vi "Test Archiver.vi"() -> ()   [LabVIEW 2019]
uses:
  Settings/Setting Database/Typedefs/PublicEvents--Setting Database.PathsUpdated.ctl
  Settings/Path Settings/Path Settings.lvclass
  C:/Users/Albro/Documents/GitHub/AFM-Lithography/lvsrc/Classes/Settings/ObjectSettings/ObjectSettings.lvclass
  Settings/Setting Database/Typedefs/PublicEvents--Setting Database.RectanglesUpdated.ctl
  Settings/Rectangle Settings/Rectangle Settings.lvclass
  Settings/Setting Database/Typedefs/PublicEvents--Setting Database.FunnelsUpdated.ctl
  Settings/Funnel Settings/Funnel Settings.lvclass
  Settings/Setting Database/Typedefs/PublicEvents--Setting Database.DotsUpdated.ctl
  Settings/Dot Settings/Dot Settings.lvclass
  Settings/Setting Database/Setting Database.lvclass
  C:/Program Files (x86)/National Instruments/LabVIEW 2019/vi.lib/JKI/JKI SMO/SMO/SMO.lvclass
  <vilib>/JKI/JKI SMO/SMO/SMO.lvclass/SMO.ctl
  <vilib>/JKI/JKI SMO/SMO/Typedefs/SMOState --Enum.ctl
  <vilib>/JKI/JKI SMO/SMO/Private/ReftoDVR--SMO.vi
  <vilib>/addons/_JKI Toolkits/Caraya/classes/Test/Test.lvclass
  <vilib>/addons/_JKI Toolkits/Caraya/classes/Assert/Assert.lvclass
  <vilib>/addons/_JKI Toolkits/Caraya/classes/Assert/Assert Equal Value_Variant.vi
  Archivist.lvclass
  <vilib>/JKI/JKI SMO/SMO/SMO.lvclass
panel:
  out "Numeric":i32
  out "GUIDs 6":string[](array[string])
  out "GUIDs 5":string[](array[string])
  out "GUIDs 4":string[](array[string])
  out "GUIDs 3":string[](array[string])
  out "GUIDs 2":string[](array[string])
  out "GUIDs":string[](array[string])
  out "number of events discarded":u32
  out "error out 2":errorcluster
  out "error out":errorcluster
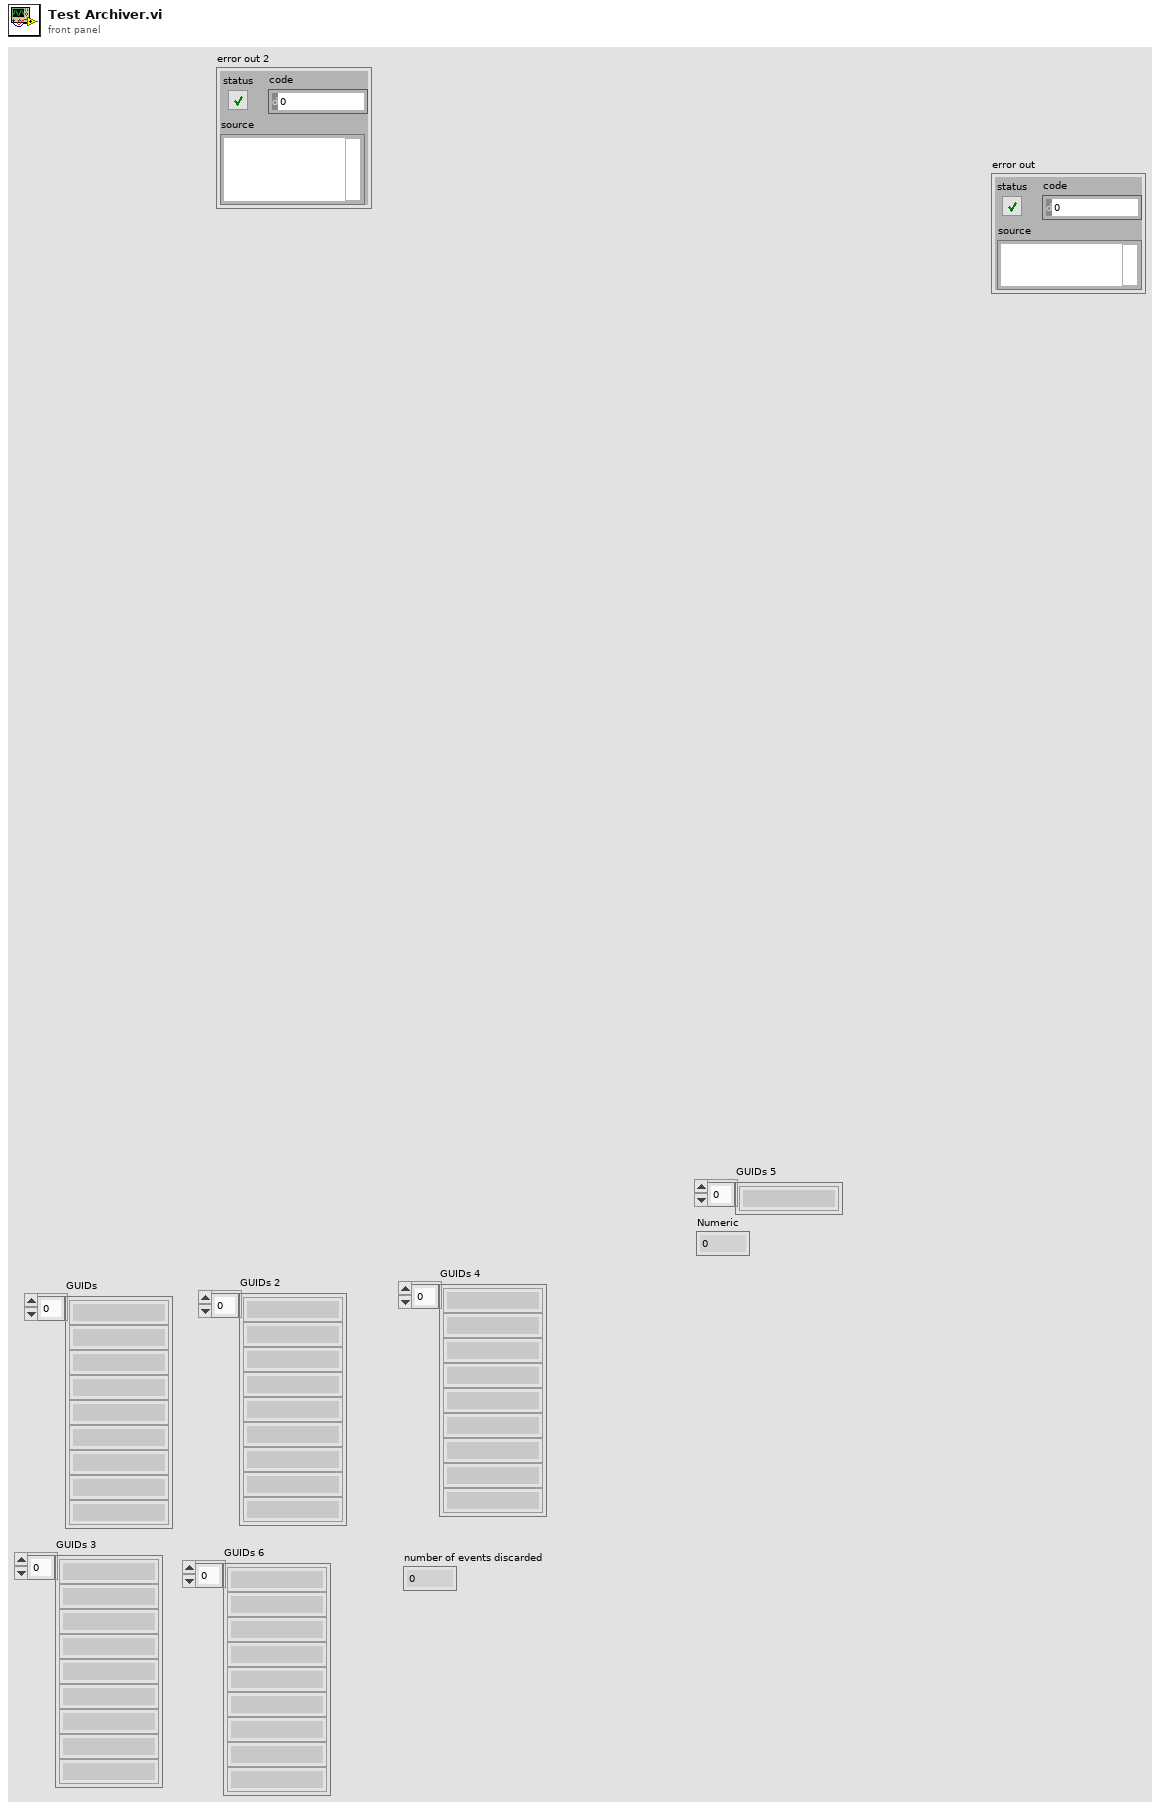
[diagram p1: front panel]
types:
  T1 = typedef "Setting Database.lvclass/PublicEvents--Setting Database.PathsUpdated.ctl" = refnum<class "Path Settings.lvclass">[]
  T2 = typedef "Setting Database.lvclass/PublicEvents--Setting Database.RectanglesUpdated.ctl" = refnum<class "Rectangle Settings.lvclass">[]
  T3 = typedef "Setting Database.lvclass/PublicEvents--Setting Database.FunnelsUpdated.ctl" = refnum<class "Funnel Settings.lvclass">[]
  T4 = typedef "Setting Database.lvclass/PublicEvents--Setting Database.DotsUpdated.ctl" = refnum<class "Dot Settings.lvclass">[]
  T5 = cluster{"Paths":T1, "Rectangles":T2, "Funnels":T3, "Dots":T4}
  T6 = typedef "Setting Database.lvclass/PublicEvents--Cluster.ctl" = cluster{"NewActivePath":refnum<user-event>, "PathsUpdated":refnum<user-event>, "RectanglesUpdated":refnum<user-event>, "NewActiveRectangle":refnum<user-event>, "NewActiveFunnel":refnum<user-event>, "FunnelsUpdated":refnum<user-event>, "NewActiveDot":refnum<user-event>, "DotsUpdated":refnum<user-event>}
  T7 = typedef "SMO.lvclass/Public Events.ctl" = cluster{"Error":refnum<user-event>, "State":refnum<user-event>, "Reserve State":refnum<user-event>}
  T8 = cluster{"Event Registration Refnum":refnum<event-registration>}
  T9 = typedef "SMO.lvclass/SMOState --Enum.ctl" = enum16{"unknown", "Created", "Started", "Stopped"}
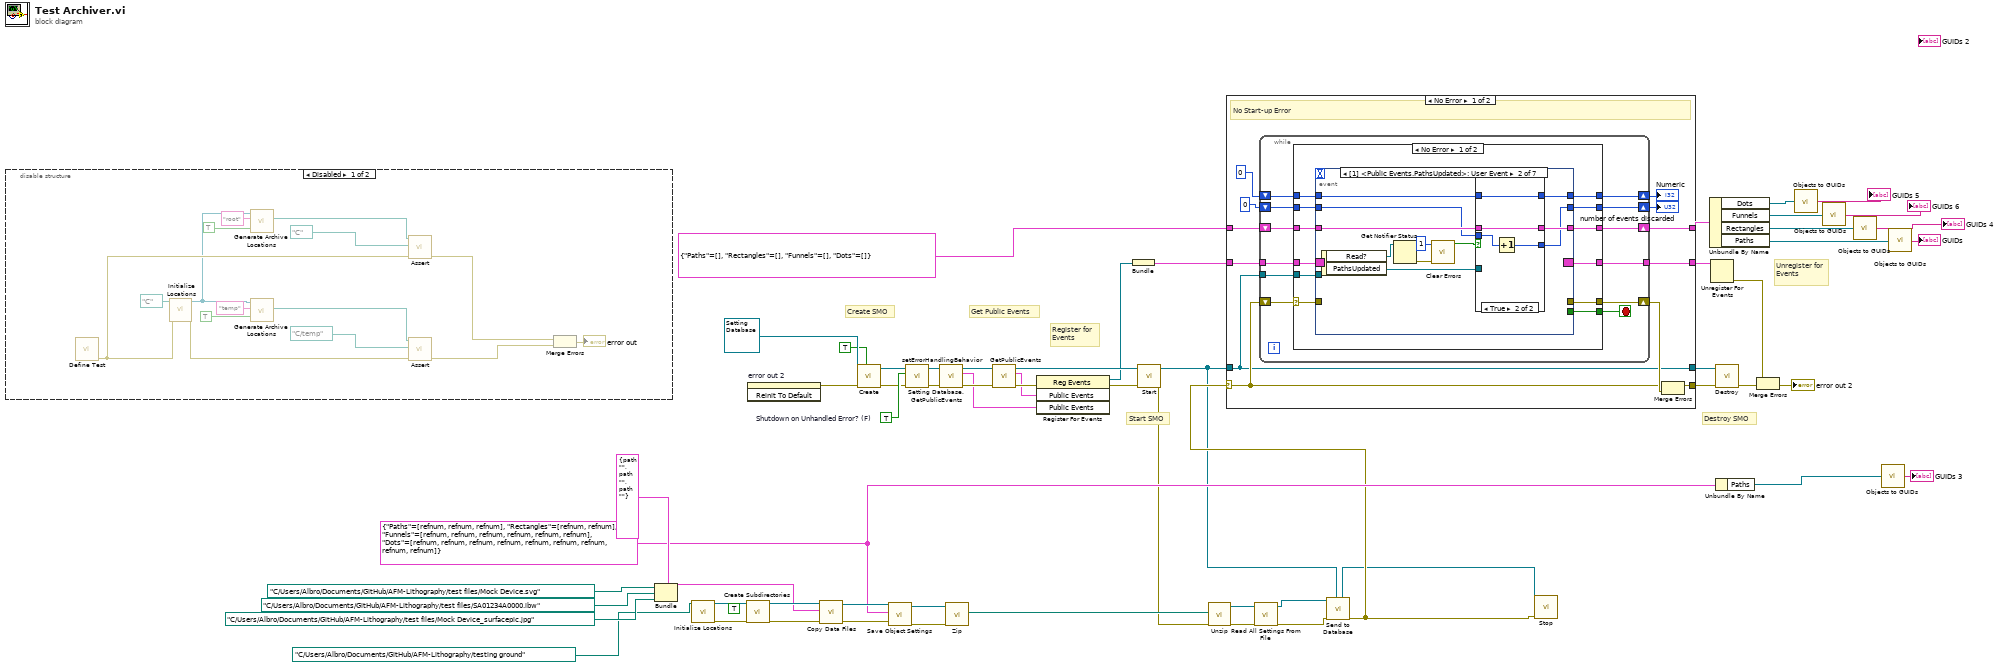
[diagram p0: block diagram]
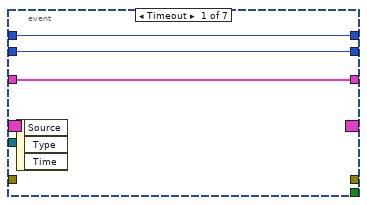
[diagram p2: hidden frame]
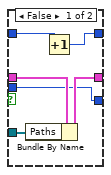
[diagram p3: hidden frame]
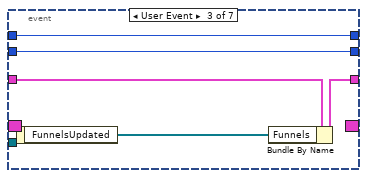
[diagram p4: hidden frame]
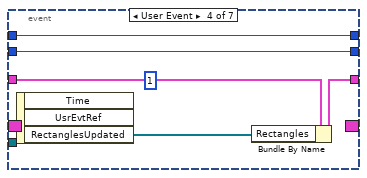
[diagram p5: hidden frame]
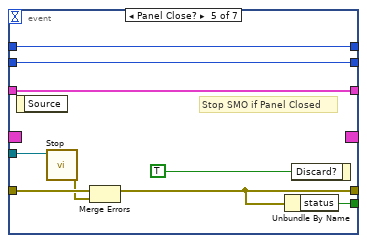
[diagram p6: hidden frame]
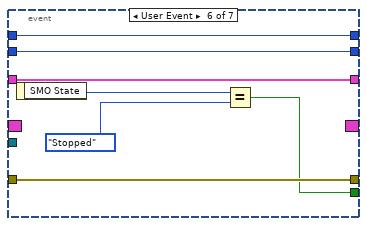
[diagram p7: hidden frame]
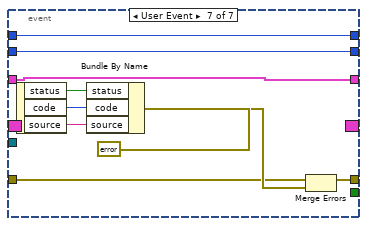
[diagram p8: hidden frame]
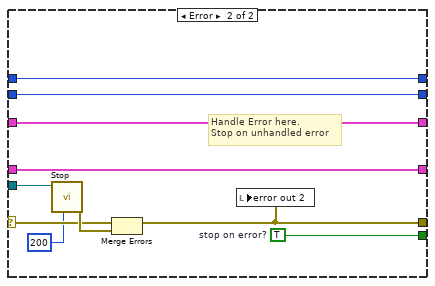
[diagram p9: hidden frame]
diagram:
  w42 = TRUE  # Shutdown on Unhandled Error? (F)
  w14 = T5 {"Paths"=[refnum, refnum, refnum], "Rectangles"=[refnum, refnum], "Funnels"=[refnum, refnum, refnum, refnum, refnum, refnum], "Dots"=[refnum, refnum, refnum, refnum, refnum, refnum, refnum, refnum, refnum]} ("Settings")
  (unwired) TRUE ("Archive?")
  # "Get Public Events"
  # "Start SMO"
  # "Destroy SMO"
  # "Create SMO"
  # "Unregister for Events"
  # "Register for Events"
  n1 = disable-structure shown="Disabled" {
    frame Disabled {
      n2 = call <vilib>:"Define Test.vi"() -> ("error out"=w64:errorcluster)  [unwired: 10 in, 1 out]
      n3 = call "Initialize Locations.vi"("error in"=w64, "Save Location"=path "C:/") -> ("error out"=w63:errorcluster, "Archivist out"=w62:refnum<class "Archivist.lvclass">)  [unwired: 8 in]
      n4 = call "Generate Archive Locations.vi"("Archive?"=TRUE, "Key"="root", "Archivist In"=w62) -> ("Path Out"=w69:path)  [unwired: 7 in, 1 out]
      n5 = call "Generate Archive Locations.vi"("Archive?"=TRUE, "Key"="temp", "Archivist In"=w62) -> ("Path Out"=w72:path)  [unwired: 7 in, 1 out]
      n6 = call-poly <vilib>:"Assert.vi"("error in (no error)"=w64, "Actual"=path "C:/", "Expected"=w69) -> ("error out"=w66:errorcluster)  [unwired: 7 in, 1 out]
      n7 = call-poly <vilib>:"Assert.vi"("error in (no error)"=w63, "Actual"=path "C:/temp", "Expected"=w72) -> ("error out"=w67:errorcluster)  [unwired: 7 in, 1 out]
      n8 = Merge Errors(w66, w67) -> (→"error out":errorcluster)
    }
    frame Enabled {
    }
  }
  n9 = Bundle(cluster=cluster{"svg":path, "afm":path, "jpg":path} {"svg"=path "", "afm"=path "", "jpg"=path ""}, "svg"=path "C:/Users/Albro/Documents/GitHub/AFM-Lithography/test files/Mock Device.svg" ("file path"), "afm"=path "C:/Users/Albro/Documents/GitHub/AFM-Lithography/test files/SA01234A0000.ibw" ("file path"), "jpg"=path "C:/Users/Albro/Documents/GitHub/AFM-Lithography/test files/Mock Device_surfacepic.jpg" ("file path")) -> (w46:cluster{"svg":path, "afm":path, "jpg":path})
  n10 = call "Initialize Locations.vi"("Save Location"=path "C:/Users/Albro/Documents/GitHub/AFM-Lithography/testing ground" ("file path")) -> ("error out"=w56:errorcluster, "Archivist out"=w59:refnum<class "Archivist.lvclass">)  [unwired: 9 in]
  n11 = call "Create Subdirectories.vi"("error in"=w56, "Archivist in"=w59) -> ("error out"=w55:errorcluster, "Archivist out"=w58:refnum<class "Archivist.lvclass">)  [unwired: 8 in]
  n12 = invoke on="error out 2" class="Clust (strict)" method="Reinit To Default"() -> (error out=w43:errorcluster)  [unwired: 3 in, 2 out]
  n13 = call "Copy Data Files.vi"("error in"=w55, "Data Files"=w46, "Archivist in"=w58) -> ("error out"=w54:errorcluster, "Archivist out"=w57:refnum<class "Archivist.lvclass">)  [unwired: 7 in]
  n14 = call <vilib>:"Create.vi"("Shared Resource (F)"=TRUE, "error in (no error)"=w43, "SMO"=refnum<class "Setting Database.lvclass"> refnum ("Setting Database.lvclass")) -> ("error out"=w41:errorcluster, "SMO out"=w40:refnum<class "Setting Database.lvclass">)  [unwired: 6 in, 1 out]
  n15 = call "Save Object Settings.vi"("error in"=w54, "Settings"=w14, "Archivist in"=w57) -> ("error out"=w52:errorcluster, "Archivist out"=w53:refnum<class "Archivist.lvclass">)  [unwired: 7 in]
  n16 = call <vilib>:"setErrorHandlingBehavior.vi"("error in (no error)"=w41, "Shutdown on Unhandled Error? (F)"=w42, "SMO in"=w40) -> ("error out"=w25:errorcluster, "SMO out"=w27:refnum<class "Setting Database.lvclass">)  [unwired: 7 in]
  n17 = call "Setting Database.GetPublicEvents.vi"("error in (no error)"=w25, "Setting Database"=w27) -> ("error out"=w24:errorcluster, "Public Events"=w23:T6, "Setting Database out"=w26:refnum<class "Setting Database.lvclass">)  [unwired: 7 in]
  n18 = call "Zip.vi"("error in"=w52, "Archivist in"=w53) -> ("archive name out"=w45:path)  [unwired: 7 in, 2 out]
  n19 = call <vilib>:"GetPublicEvents.vi"("error in (no error)"=w24, "SMO"=w26) -> ("error out"=w38:errorcluster, "Public Events"=w37:T7, "SMO out"=w44:refnum<class "Setting Database.lvclass">)  [unwired: 7 in]
  n20 = register-events(error in=w38, w37, w23) -> (reference out=w35:refnum<event-registration>, error out=w36:errorcluster)  [unwired: 1 in]
  n21 = Bundle("Event Registration Refnum"=w35) -> (w31:T8)  [unwired: 1 in]
  n22 = call <vilib>:"Start.vi"("error in (no error)"=w36, "SMO"=w44) -> ("error out"=w5:errorcluster, "SMO out"=w3:refnum<class "Setting Database.lvclass">)  [unwired: 8 in]
  n23 = call "Unzip.vi"("error in"=w5, "Path"=w45) -> ("error out"=w17:errorcluster, "Archivist out"=w18:refnum<class "Archivist.lvclass">)  [unwired: 8 in]
  n24 = call "Read All Settings From File.vi"("error in"=w17, "Archivist in"=w18) -> ("error out"=w16:errorcluster, "Archivist out"=w1:refnum<class "Archivist.lvclass">)  [unwired: 8 in]
  n25 = call "Send to Database.vi"("Setting Database In"=w3, "error in"=w16, "Archivist in"=w1) -> ("error out"=w4:errorcluster, "Setting Database Out"=w2:refnum<class "Setting Database.lvclass">)  [unwired: 6 in, 1 out]
  n26 = case shown="No Error" w4 {
    selector: w4 -> [w82 w183]
    tunnel: [w86 w184] -> w30
    tunnel: w31 -> [w85 w184]
    tunnel: [w83 w183] -> w39
    tunnel: w3 -> [w81 w182]
    tunnel: [w81 w182] -> w15
    tunnel: T5 {"Paths"=[], "Rectangles"=[], "Funnels"=[], "Dots"=[]} ("Settings") -> [w80 w181]
    tunnel: [w79 w181] -> w22
    frame No Error {
      # "No Start-up Error"
      n27 = while {
        shift-right: [w97] -> w84
        shift-left: w82 -> [w93]
        tunnel: w85 -> [w96]
        tunnel: [w95] -> w86
        tunnel: w81 -> [w94]
        shift-right: [w91] -> w79
        shift-left: w80 -> [w92]
        shift-right: [w89] -> w78
        shift-left: 0 -> [w90]
        shift-right: [w88] -> w75
        shift-left: 0 -> [w87]
        stop <- w98 stop-if-true
        n28 = case shown="No Error" w93 {
          selector: w93 -> [w105 w177]
          tunnel: [w110 w180] -> w98
          tunnel: [w109 w174] -> w97
          tunnel: w96 -> [w108 w179]
          tunnel: [w107 w179] -> w95
          tunnel: w94 -> [w106 w176]
          tunnel: w92 -> [w104 w173]
          tunnel: [w103 w173] -> w91
          tunnel: w90 -> [w102 w172]
          tunnel: [w101 w172] -> w89
          tunnel: w87 -> [w99 w171]
          tunnel: [w100 w171] -> w88
          frame No Error {
            n29 = event shown="[1] <Public Events.PathsUpdated>: User Event" {
              selector: w108 -> [_ _ _ _ _ _ _]
              dyn-events: [_ _ _ _ _ _ _] -> w107
              timeout: _ -> [_ _ _ _ _ _ _]
              tunnel: [_ _ _ _ w151 w157 _] -> w110
              tunnel: w106 -> [_ _ _ _ w153 _ _]
              tunnel: [_ _ _ _ w148 w158 w164] -> w109
              tunnel: w105 -> [_ _ _ _ w150 w158 w165]
              tunnel: w104 -> [w113 w123 w138 w142 w147 w156 w163]
              tunnel: [w113 w124 w139 w144 w147 w156 w163] -> w103
              tunnel: w102 -> [w112 w116 w136 w141 w146 w155 w162]
              tunnel: [w112 w117 w136 w141 w146 w155 w162] -> w101
              tunnel: w99 -> [w111 w115 w135 w140 w145 w154 w161]
              tunnel: [w111 w114 w135 w140 w145 w154 w161] -> w100
              event Timeout {
                n30 = event-data() -> ()  [unwired: 1 in, 3 out]
              }
              event User Event {
                n31 = event-data() -> ("Read?"=w121:refnum<notifier>, "PathsUpdated"=w122:T1)  [unwired: 1 in]
                n32 = Get Notifier Status(notifier=w121) -> (error out=w120:errorcluster)  [unwired: 1 in, 4 out]
                n33 = call <vilib>:"Clear Errors.vi"("error in (no error)"=w120, "specific error code to clear (0: all)"=1) -> ("specific error cleared?"=w118:bool)  [unwired: 4 in, 1 out]
                n34 = case shown="True" w118 {
                  tunnel: [w130 w134] -> w124
                  tunnel: w123 -> [w129 w134]
                  tunnel: w122 -> [w128 _]
                  tunnel: w116 -> [w127 w133]
                  tunnel: [w127 w132] -> w117
                  tunnel: w115 -> [w125 w131]
                  tunnel: [w126 w131] -> w114
                  frame False {
                    n35 = Bundle By Name(cluster=w129, "Paths"=w128) -> (w130:T5)
                    n36 = Increment(x=w125) -> (x+1=w126:i32)
                  }
                  frame True {
                    n37 = Increment(x=w133) -> (x+1=w132:i32)
                  }
                }
              }
              event User Event {
                n38 = event-data() -> ("FunnelsUpdated"=w137:T3)  [unwired: 1 in]
                n39 = Bundle By Name(cluster=w138, "Funnels"=w137) -> (w139:T5)
              }
              event User Event {
                (unwired) 1 ("keep most recent")
                n40 = event-data() -> ("RectanglesUpdated"=w143:T2)  [unwired: 1 in, 2 out]
                n41 = Bundle By Name(cluster=w142, "Rectangles"=w143) -> (w144:T5)
              }
              event Panel Close? {
                # "Stop SMO if Panel Closed"
                n42 = event-data() -> ()  [unwired: 1 in, 1 out]
                n43 = call <vilib>:"Stop.vi"("SMO"=w153) -> ("error out"=w149:errorcluster)  [unwired: 9 in, 1 out]
                n44 = Merge Errors(w150, w149) -> (w148:errorcluster)
                n45 = Unbundle By Name(w148) -> ("status"=w151:bool)
                n46 = event-data("Discard?"=TRUE ("OK")) -> ()  [unwired: 1 in, 1 out]
              }
              event User Event {
                n47 = event-data() -> ("SMO State"=w160:T9)  [unwired: 1 in]
                n48 = Equal?(x=w160, y=SMOState_--Enum."Stopped") -> (x = y?=w157:bool)
              }
              event User Event {
                n49 = event-data() -> ("status"=w170:bool, "code"=w169:i32, "source"=w168:string)  [unwired: 1 in]
                n50 = Bundle By Name(cluster=errorcluster {"status"=FALSE, "code"=0, "source"=""} ("error out"), "status"=w170, "code"=w169, "source"=w168) -> (w166:errorcluster)
                n51 = Merge Errors(w165, w166) -> (w164:errorcluster)
              }
            }
          }
          frame Error {
            w180 = TRUE  # stop on error?
            # "Handle Error here.\nStop on unhandled error"
            n52 = call <vilib>:"Stop.vi"("timeout in ms (-1)"=200, "SMO"=w176) -> ("error out"=w178:errorcluster)  [unwired: 8 in, 1 out]
            n53 = Merge Errors(w177, w178) -> (w174:errorcluster)
            n54 = local write "error out 2"(w174) -> ()
          }
        }
      }
      "number of events discarded" <- w78
      "Numeric" <- w75
      n55 = Merge Errors(w82, w84) -> (w83:errorcluster)
    }
    frame Error {
      # "Error occured before starting the process"
    }
  }
  n56 = call <vilib>:"Stop.vi"("error in (no error)"=w4, "SMO"=w2) -> ()  [unwired: 8 in, 2 out]
  n57 = Unbundle By Name(w22) -> ("Dots"=w8:T4, "Funnels"=w9:T3, "Rectangles"=w10:T2, "Paths"=w20:T1)
  n58 = Unregister For Events(event registration refnum=w30) -> (error out=w32:errorcluster)  [unwired: 1 in]
  n59 = call <vilib>:"Destroy.vi"("error in (no error)"=w39, "SMO"=w15) -> ("error out"=w34:errorcluster)  [unwired: 9 in]
  n60 = Unbundle By Name(w14) -> ("Paths"=w12:T1)
  n61 = Merge Errors(w32, w34) -> (→"error out 2":errorcluster)
  n62 = call "Objects to GUIDs.vi"("Objects"=w8) -> ("GUIDs"=→"GUIDs 5":string[])  [unwired: 3 in, 1 out]
  n63 = call "Objects to GUIDs.vi"("Objects"=w9) -> ("GUIDs"=→"GUIDs 6":string[])  [unwired: 3 in, 1 out]
  n64 = call "Objects to GUIDs.vi"("Objects"=w10) -> ("GUIDs"=→"GUIDs 4":string[])  [unwired: 3 in, 1 out]
  n65 = call "Objects to GUIDs.vi"("Objects"=w12) -> ("GUIDs"=→"GUIDs 3":string[])  [unwired: 3 in, 1 out]
  n66 = call "Objects to GUIDs.vi"("Objects"=w20) -> ("GUIDs"=→"GUIDs":string[])  [unwired: 3 in, 1 out]
